vi "Populate Tree.vi"(8 "error in (no error)":errorcluster, 9 "VI Properties":T1[](array[typedef]), 10 "Tree Refnum":refnum<vi>, 11 "Project in":refnum<vi>) -> (0 "error out":errorcluster, 3 "Project out":refnum<vi>)   [LabVIEW 2019, in "Project Properties.lvlib"]
doc: "Populates the Project Explorer Tree control with the <b>VI Properties</b> specified.\n\nCreated by: Ryan Pacini"
uses:
  Project Properties.lvlib
  VI Property.ctl
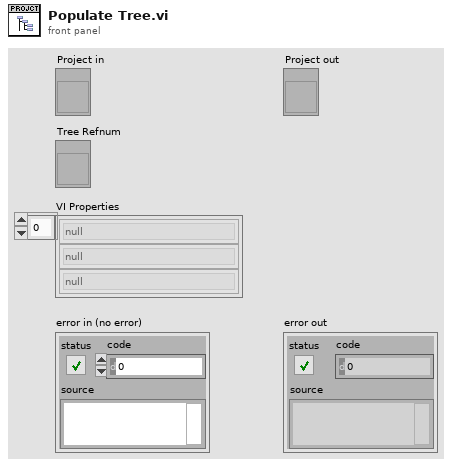
[diagram p1: front panel]
types:
  T1 = typedef "Project Properties.lvlib/VI Property.ctl" = enum8{"null", "Auto Logging:Log at Finish", "Auto Logging:Log File Path", "Auto Logging:Print at Finish", "Auto Preallocate Arrays and Strings", "Automatic Error Handling", "BD Master Wizard", "Block Diagram", "Block Diagram Window:Alignment Grid Size", "Block Diagram Window:Native Window", "Block Diagram Window:Open", "Block Diagram Window:Origin", "Block Diagram Window:State", "Block Diagram Window:Window Bounds", "Block Diagram Window:Window Interface", "Callers' Names", "Callers' Paths", "Compiled:Code Complexity", "Compiled:Last Compiled With", "Compiler:Generated Code Profiling Result", "Compiler:Generated Code Profiling Settings", "Connector Pane:Checksum Ignore Dynamic Dispatch v2", "Connector Pane:Checksum v3", "Connector Pane:DataType", "Connector Pane:Reference", "Connector Pane:Set", "Contains Compiled Code", "Context:Has Edits In Another Context", "Context:Has Edits In This Context", "Context:Is Reserved In Other Context", "Context:Is Reserved In This Context", "Control VI Type", "Did Recompile InThis Version", "Do Not Show Save Changes Dialog", "Edit Mode On Open", "Execution highlighting?", "Execution:Allow Debugging", "Execution:Close After Call", "Execution:Compiled With SSE", "Execution:Did Compiler Or User Approve Inlining", "Execution:Inline Enum", "Execution:Inline Is Allowed", "Execution:Inline SubVI", "Execution:Inline SubVI If Possible", "Execution:Is Reentrant", "Execution:Preferred Exec System", "Execution:Priority", "Execution:Reentrancy Type", "Execution:Retain Wire Values", "Execution:Run When Opened", "Execution:Show Front Panel On Call", "Execution:Show Front Panel On Load", "Execution:Shrink Large Buffer Threshold", "Execution:Shrink Large Buffers", "Execution:SSE Runtime Optimization", "Execution:State", "Execution:Suspend On Call", "Expand When Dropped As SubVI", "Front Panel", "Front Panel RefNum TD", "Front Panel Window:Alignment Grid Size", "Front Panel Window:Allow Runtime PopUp", "Front Panel Window:Behavior", "Front Panel Window:Closeable", "Front Panel Window:Custom Title", "Front Panel Window:Highlight Return Button", "Front Panel Window:Is Floating", "Front Panel Window:Is Frontmost", "Front Panel Window:Keep Window Proportions", "Front Panel Window:Minimizable", "Front Panel Window:Minimum Size", "Front Panel Window:Monitor", "Front Panel Window:Native Window", "Front Panel Window:Panel Bounds", "Front Panel Window:Resizable", "Front Panel Window:Run VI Transparently", "Front Panel Window:Show Menu Bar", "Front Panel Window:State", "Front Panel Window:Title", "Front Panel Window:Title Bar Visible", "Front Panel Window:Transparency", "Front Panel Window:Window Bounds", "Front Panel Window:Window Interface", "Has MathScript Nodes", "Help:Document Path", "Help:Document Tag", "Help:Document Web URL", "Help:Examples Exist", "Help:Use Web URL", "Hide Instance VI Caption On Drop", "History:Always Add Comments At Save", "History:Entire Text", "History:Prompt for Comments At Close", "History:Prompt for Comments At Save", "History:Record Application Comments", "History:Revision Number", "History:Use Defaults", "Inline Callees", "Is Clone VI", "Is Generic", "Is In Packed Library", "Is Instance", "Is Probe", "Is Running Interactively", "Is Skinned", "Is System VI", "Is VI Paused?", "Is XNode VI", "Item ID", "Ladder VI Needs Scripting", "Library", "Library:Private", "Library:Version", "Metrics:Advanced", "Metrics:Block Diagram Loaded", "Metrics:Code Size", "Metrics:Front Panel Loaded", "Metrics:Number of clones", "Metrics:Size of Block Diagram", "Metrics:Size of Front Panel", "Metrics:Total Data Size", "Modifications:Block Diagram Mods Bitset", "Modifications:Front Panel Mods Bitset", "Modifications:User Changes", "Modifications:VI Modifications Bitset", "Modifications:VI Signatures", "Modifications:VI User Code GUID", "No Clone If Instance VI", "Number of Non-Proxy Callers", "Overload Info", "Owning Application", "Printing:Block Diagram Scaling?", "Printing:Front Panel Scaling?", "Printing:Header Content:Date Printed?", "Printing:Header Content:Modify Date?", "Printing:Header Content:Page Number?", "Printing:Header Content:VI Icon?", "Printing:Header Content:VI Name?", "Printing:Header Content:VI Path?", "Printing:Margins", "Printing:Page Headers?", "Printing:Page Orientation", "Purgative", "Run-Time Menu Path", "Saved Version", "Statechart:Is Sub Panel Editable", "Statechart:Supress Parse", "Suppress Data Manager", "Suppress Instance VI Halo", "Suppress Transact Info", "Suppress Type Prop", "Tagged And Not Edited", "Terminal Bounds[]", "Tool Bar:Show Abort Button", "Tool Bar:Show Free Run Button", "Tool Bar:Show Run Button", "Tool Bar:Visible", "Tool Kit Attr", "VI Clone Name", "VI Compile Time", "VI Description", "VI Linker Errors", "VI Name", "VI Path", "VI Type"}
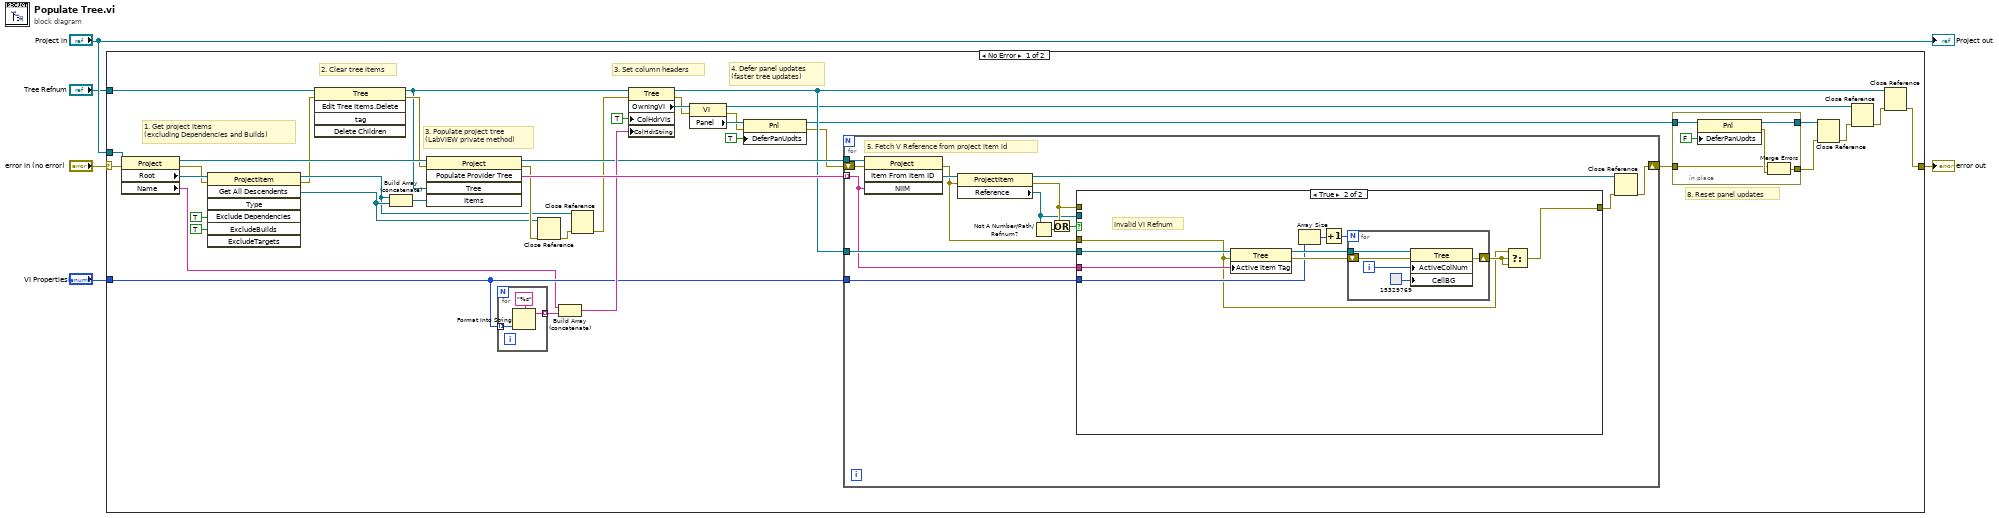
[diagram p0: block diagram]
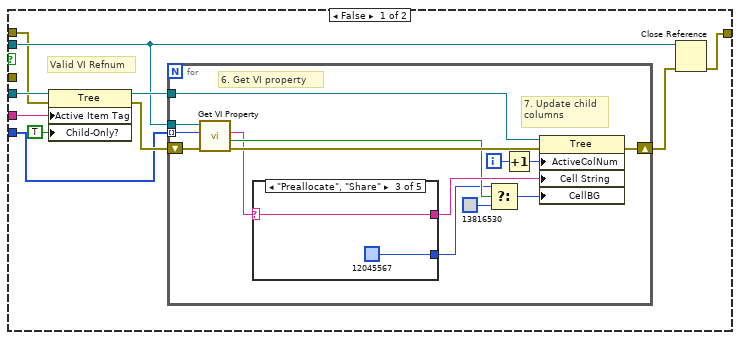
[diagram p2: hidden frame]
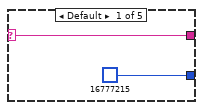
[diagram p3: hidden frame]
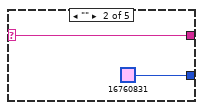
[diagram p4: hidden frame]
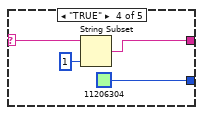
[diagram p5: hidden frame]
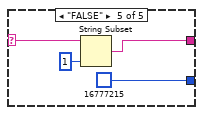
[diagram p6: hidden frame]
diagram:
  n1 = case shown="No Error" "error in (no error)" {
    selector: "error in (no error)" -> [w10 w121]
    tunnel: "Project in" -> [w9 _]
    tunnel: [w8 w121] -> w3
    tunnel: "Tree Refnum" -> [w14 _]
    tunnel: "VI Properties" -> [w37 _]
    frame No Error {
      # "8. Reset panel updates"
      # "4. Defer panel updates\n(faster tree updates)"
      # "3. Set column headers"
      # "3. Populate project tree\n(LabVIEW private method)"
      # "2. Clear tree items"
      # "1. Get project items\n(excluding Dependencies and Builds)"
      n2 = property class="Project"(reference=w9, error in=w10) -> (reference out=w44:refnum<vi>, error out=w35:errorcluster, "Root"=w36:refnum<vi>, "Name"=w6:string)
      n3 = invoke class="ProjectItem" method="Get All Descendents"(reference=w36, error in=w35, "Exclude Dependencies"=TRUE ("ExcludeDependencies"), "ExcludeBuilds"=TRUE) -> (reference out=w15:refnum<vi>, error out=w13:errorcluster, "All Descendents"=w16:refnum<vi>[])  [unwired: 3 in, 4 out]
      n4 = invoke class="Tree" method="Edit Tree Items.Delete"(reference=w14, error in=w13) -> (reference out=w11:refnum<vi>, error out=w12:errorcluster)  [unwired: 3 in, 3 out]
      n5 = Build Array (concatenate)(w15, w16) -> (w30:refnum<vi>[])
      n6 = invoke class="Project" method="Populate Provider Tree"(reference=w44, error in=w12, "Tree"=w11, "Items"=w30) -> (reference out=w39:refnum<vi>, error out=w18:errorcluster, "Populate Provider Tree"=w42:string[])  [unwired: 1 in, 2 out]
      n7 = for {
        tunnel: w37 -> [w53] mode=indexing
        tunnel: [w51] -> w43 mode=indexing
        n8 = Format Into String(format string="%s", w53) -> (resulting string=w51:string)  [unwired: 2 in, 1 out]
      }
      n9 = Close Reference(reference=w16, error in (no error)=w18) -> (error out=w19:errorcluster)
      n10 = Build Array (concatenate)(w6, w43) -> (w41:string[])
      n11 = Close Reference(reference=w15, error in (no error)=w19) -> (error out=w17:errorcluster)
      n12 = property class="Tree"(reference=w11, error in=w17, "ColHdrVis"=TRUE ("Visible Items:Column Headers Visible"), "ColHdrString"=w41) -> (reference out=w38:refnum<vi>, error out=w27:errorcluster, "OwningVI"=w31:refnum<vi>)
      n13 = property class="VI"(reference=w31, error in=w27) -> (reference out=w20:refnum<vi>, error out=w29:errorcluster, "Panel"=w32:refnum<vi>)
      n14 = property class="Pnl"(reference=w32, error in=w29, "DeferPanUpdts"=TRUE ("Defer Panel Updates")) -> (reference out=w24:refnum<vi>, error out=w26:errorcluster)
      n15 = for {
        tunnel: w39 -> [w66]
        tunnel: w42 -> [w56] mode=indexing
        shift-right: [w55] -> w7
        shift-left: w26 -> [w67]
        tunnel: w37 -> [w64]
        tunnel: w38 -> [w57]
        # "5. Fetch V Reference from project item id"
        n16 = invoke class="Project" method="Item From Item ID"(reference=w66, error in=w67, "NIIM"=w56) -> (error out=w58:errorcluster, "GetItemFromNIIM"=w65:refnum<vi>)  [unwired: 1 in, 2 out]
        n17 = property class="ProjectItem"(reference=w65, error in=w58) -> (reference out=w54:refnum<vi>, error out=w63:errorcluster, "Reference"=w62:refnum<vi>)
        n18 = Not A Number/Path/Refnum?(number/path/refnum=w62) -> (NaN/Path/Refnum?=w61:bool)
        n19 = Or(x=w63, y=w61) -> (x .or. y?=w59:bool)
        n20 = case shown="True" w59 {
          tunnel: w64 -> [w69 w111]
          tunnel: w63 -> [w70 _]
          tunnel: w62 -> [w72 _]
          tunnel: [w76 w107] -> w60
          tunnel: w58 -> [_ w108]
          tunnel: w57 -> [w74 w115]
          tunnel: w56 -> [w73 w114]
          frame False {
            # "Valid VI Refnum"
            n21 = property class="Tree"(reference=w74, error in=w70, "Active Item Tag"=w73, "Child-Only?"=TRUE ("Active Item:Child-Only?")) -> (reference out=w75:refnum<vi>, error out=w71:errorcluster)
            n22 = for {
              tunnel: w72 -> [w90]
              tunnel: w69 -> [w89] mode=indexing
              shift-right: [w85] -> w77
              shift-left: w71 -> [w91]
              tunnel: w75 -> [w79]
              i -> [w88]
              # "7. Update child\ncolumns"
              # "6. Get VI property"
              n23 = call "Get VI Property.vi"("error in (no error)"=w91, "VI Property"=w89, "VI Refnum in"=w90) -> ("error out"=w86:errorcluster, "Supported?"=w83:bool, "Value"=w78:string)  [unwired: 5 in, 1 out]
              n24 = case shown="\"Preallocate\", \"Share\"" w78 {
                selector: w78 -> [w93 w95 w97 w101 w105]
                tunnel: [w93 w95 w97 w100 w104] -> w84
                tunnel: [u32 16777215 u32 16760831 u32 12045567 u32 11206304 u32 16777215] -> w82
                frame Default {
                }
                frame "" {
                }
                frame "Preallocate", "Share" {
                }
                frame "TRUE" {
                  n25 = String Subset(string=w101, length (rest)=1 ("length (rest)")) -> (substring=w100:string)  [unwired: 1 in]
                }
                frame "FALSE" {
                  n26 = String Subset(string=w105, length (rest)=1 ("length (rest)")) -> (substring=w104:string)  [unwired: 1 in]
                }
              }
              n27 = Select(t=w82, s=w83, f=u32 13816530) -> (s? t:f=w80:u32)
              n28 = Increment(x=w88) -> (x+1=w87:i32)
              n29 = property class="Tree"(reference=w79, error in=w86, "ActiveColNum"=w87, "Cell String"=w84, "CellBG"=w80) -> (error out=w85:errorcluster)  [unwired: 1 out]
            }
            n30 = Close Reference(reference=w72, error in (no error)=w77) -> (error out=w76:errorcluster)
          }
          frame True {
            # "Invalid VI Refnum"
            n31 = property class="Tree"(reference=w115, error in=w108, "Active Item Tag"=w114) -> (reference out=w113:refnum<vi>, error out=w112:errorcluster)
            n32 = Array Size(array=w111) -> (size(s)=w110:i32)
            n33 = Increment(x=w110) -> (x+1=w106:i32)
            n34 = for {
              N: w106 -> [_]
              tunnel: w113 -> [w120]
              shift-right: [w117] -> w109
              shift-left: w112 -> [w119]
              i -> [w116]
              n35 = property class="Tree"(reference=w120, error in=w119, "ActiveColNum"=w116, "CellBG"=u32 15329769) -> (error out=w117:errorcluster)  [unwired: 1 out]
            }
            n36 = Select(t=w108, s=w109, f=w109) -> (s? t:f=w107:errorcluster)
          }
        }
        n37 = Close Reference(reference=w54, error in (no error)=w60) -> (error out=w55:errorcluster)
      }
      n38 = in-place {
        in-place-border: [w46] -> w25
        in-place-border: w24 -> [w48]
        in-place-border: [w47] -> w22
        in-place-border: w7 -> [w45]
        n39 = property class="Pnl"(reference=w48, "DeferPanUpdts"=FALSE ("Defer Panel Updates")) -> (reference out=w47:refnum<vi>, error out=w49:errorcluster)  [unwired: 1 in]
        n40 = Merge Errors(w45, w49) -> (w46:errorcluster)
      }
      n41 = Close Reference(reference=w22, error in (no error)=w25) -> (error out=w23:errorcluster)
      n42 = Close Reference(reference=w20, error in (no error)=w23) -> (error out=w21:errorcluster)
      n43 = Close Reference(reference=w38, error in (no error)=w21) -> (error out=w8:errorcluster)
    }
    frame Error {
    }
  }
  "error out" <- w3
  "Project out" <- "Project in"
